vi "保存功率控制表和标定参数表.vi"(7 "SN":string, 8 "功率控制表":refnum<vi>, 9 "标定参数表":refnum<vi>, 11 "该应用程序":refnum<vi>) -> ()   [LabVIEW 2015]
uses:
  <vilib>/addons/_office/excel.llb/Excel Easy Table (str).vi
  <vilib>/Utility/NIReport.llb/NI_report.lvclass
  <vilib>/Utility/NIReport.llb/Excel/NI_Excel.lvclass
  <vilib>/addons/_office/NI_ReportGenerationToolkit.lvlib
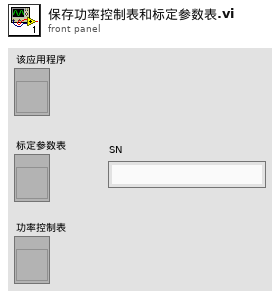
[diagram p1: front panel]
types:
  T1 = enum16{"Standard Report", "HTML", "Word", "Excel"}
  T2 = enum16{"maximized", "minimized", "normal", "no change"}
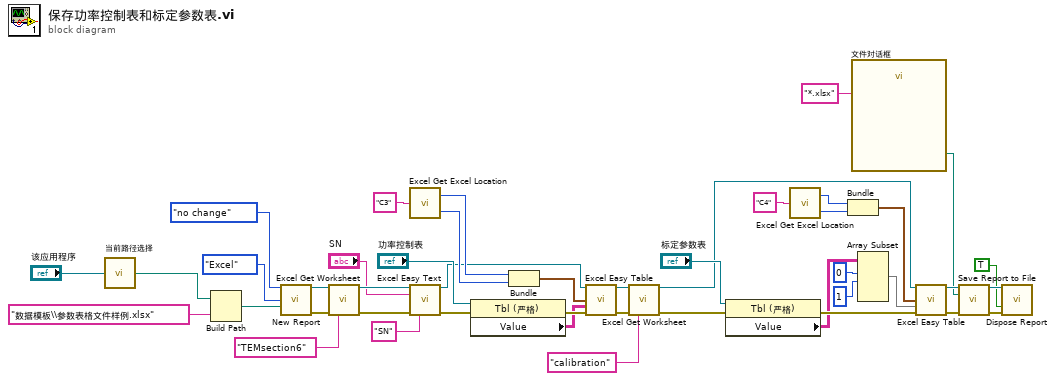
[diagram p0: block diagram]
diagram:
  n1 = call "当前路径选择.vi"("本应用程序"="该应用程序") -> ("当前路径"=w37:path)
  n2 = Build Path(base path=w37, name or relative path="数据模板\\参数表格文件样例.xlsx" ("名称或相对路径")) -> (appended path=w36:path)
  n3 = call <vilib>:"New Report.vi"("window state (normal)"=T2."no change", "report type"=T1."Excel", "template (empty)"=w36) -> ("report out"=w35:refnum<class "NI_report.lvclass">, "error out"=w34:errorcluster)  [unwired: 11 in]
  n4 = call <vilib>:"Excel Get Worksheet.vi"("report in"=w35, "error in (no error)"=w34, "name (\"\")"="TEMsection6" ("name (\"\")")) -> ("report out"=w25:refnum<class "NI_report.lvclass">, "error out"=w26:errorcluster)  [unwired: 11 in]
  n5 = call <vilib>:"Excel Get Excel Location.vi"("cell's name"="C3") -> ("row"=w31:i32, "column"=w30:i32)
  n6 = call <vilib>:"Excel Easy Text.vi"("report in"=w25, "text"="SN", "error in (no error)"=w26, "name (\"\")"="SN" ("name (\"\")")) -> ("report out"=w20:refnum<class "NI_report.lvclass">, "error out"=w22:errorcluster)  [unwired: 7 in, 3 out]
  n7 = property class="Tbl (严格)"(reference="功率控制表", error in=w22) -> (error out=w21:errorcluster, "Value"=w19:string[][])  [unwired: 1 out]
  n8 = Bundle("row"=w31, "column"=w30) -> (w18:cluster{"row":i32, "column":i32})  [unwired: 1 in]
  n9 = call-poly <vilib>:"Excel Easy Table.vi"("report in"=w20, "start (0, 0)"=w18, "text data"=w19, "error in (no error)"=w21) -> ("report out"=w17:refnum<class "NI_report.lvclass">, "error out"=w16:errorcluster)  [unwired: 7 in, 3 out]
  n10 = call <vilib>:"Excel Get Worksheet.vi"("report in"=w17, "error in (no error)"=w16, "name (\"\")"="calibration" ("name (\"\")")) -> ("report out"=w14:refnum<class "NI_report.lvclass">, "error out"=w1:errorcluster)  [unwired: 11 in]
  n11 = property class="Tbl (严格)"(reference="标定参数表", error in=w1) -> (error out=w15:errorcluster, "Value"=w13:string[][])  [unwired: 1 out]
  n12 = call <vilib>:"Excel Get Excel Location.vi"("cell's name"="C4") -> ("row"=w43:i32, "column"=w44:i32)
  n13 = Bundle("row"=w43, "column"=w44) -> (w9:cluster{"row":i32, "column":i32})  [unwired: 1 in]
  n14 = call "文件对话框"("pattern (all files)"="*.xlsx") -> ("selected path"=w6:path)  [unwired: 11 in, 3 out]
  n15 = Array Subset(array=w13, index (row)=0 ("索引 (行)"), length (row)=1 ("索引 (行)")) -> (w10:string[][])  [unwired: 2 in]
  n16 = call-poly <vilib>:"Excel Easy Table.vi"("report in"=w14, "start (0, 0)"=w9, "text data"=w10, "error in (no error)"=w15) -> ("report out"=w7:refnum<class "NI_report.lvclass">, "error out"=w8:errorcluster)  [unwired: 7 in, 3 out]
  n17 = call-dynamic "Save Report to File.vi"("report in"=w7, "report file path"=w6, "error in (no error)"=w8) -> ("report out"=w4:refnum<class "NI_report.lvclass">, "error out"=w5:errorcluster)  [unwired: 11 in]
  n18 = call-dynamic "Dispose Report.vi"("report in"=w4, "save changes? (F)"=TRUE, "error in (no error)"=w5) -> ()  [unwired: 12 in, 1 out]
